vi "Save multiple images with metadata to new tiff stack.vi"(4 "ImageDescriptions":string[](array[string]), 5 "Add metadata? (T)":bool=TRUE, 6 "Show Progress? (T)":bool=TRUE, 7 "Compression Type (None)":i32(ring) items=["None", "JPEG", "Run Length Encoded", "Zip"], 8 "error in":errorcluster, 9 "Convert to U16?":bool, 10 "Array of Images (U8, U16, I16)":T1[](array[typedef]), 11 "Path":path) -> (0 "error out":errorcluster)   [LabVIEW 2013, in "Tiff reader.lvlib"]
doc: "This .vi saves an array of images into a new single .tiff stack file."
uses:
  Tiff reader.lvlib
  <vilib>/vision/Image Controls.llb/IMAQ Image.ctl
  <vilib>/vision/NI_Vision_Development_Module.lvlib
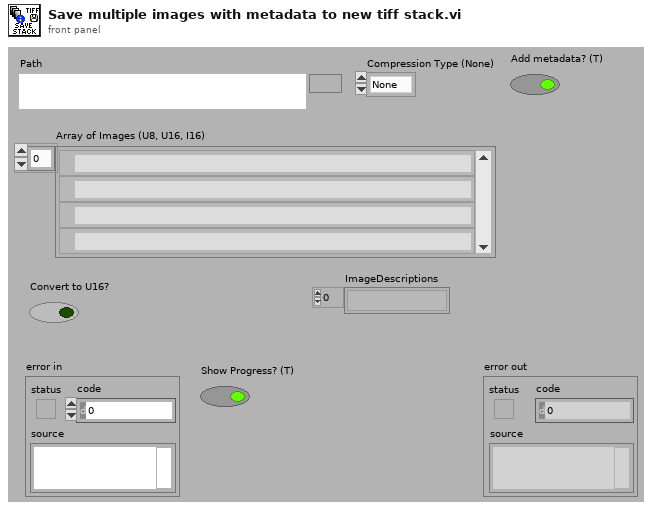
[diagram p1: front panel]
types:
  T1 = typedef "IMAQ Image.ctl" = refnum<image>
  T2 = cluster{"Rows Per Strip":i32, "Photometric":i32, "Compression Type":i32}
  T3 = typedef "Image Type" = u32
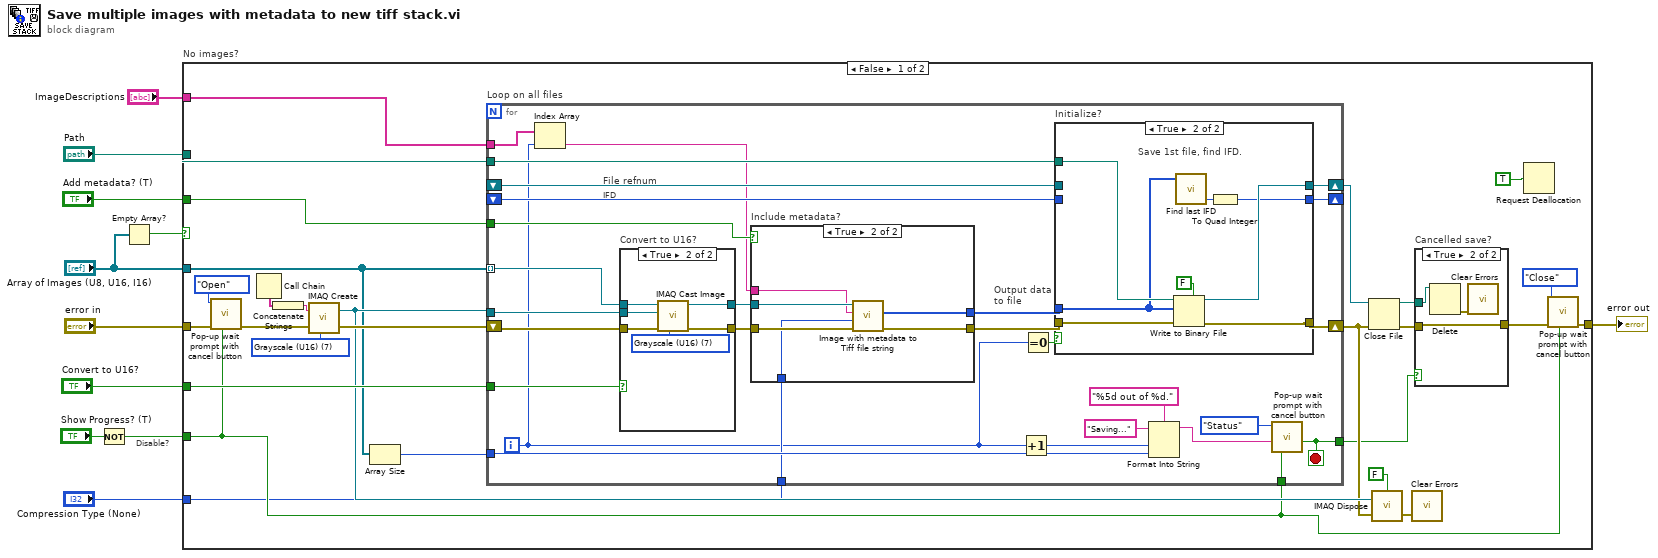
[diagram p0: block diagram]
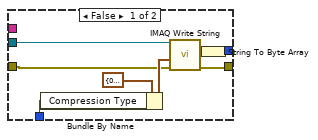
[diagram p3: hidden frame]
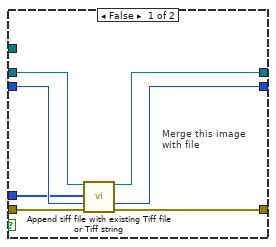
[diagram p5: hidden frame]
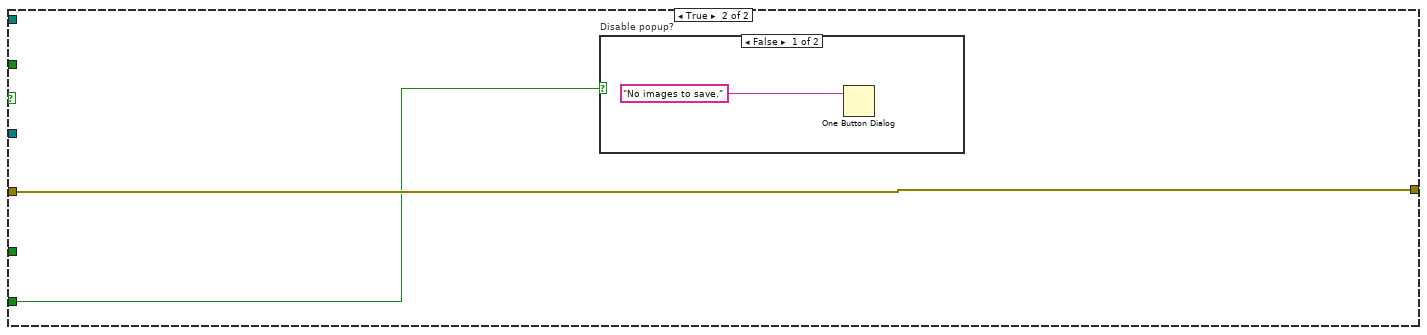
[diagram p6: hidden frame]
diagram:
  # "Disable?"
  n1 = Not(x="Show Progress? (T)") -> (.not. x?=w4:bool)
  n2 = Empty Array?(array="Array of Images (U8, U16, I16)") -> (empty?=w7:bool)
  n3 = case "No images?" shown="False" w7 {
    tunnel: "Array of Images (U8, U16, I16)" -> [w26 _]
    tunnel: [w38 w109] -> w10
    tunnel: "error in" -> [w35 w109]
    tunnel: "Path" -> [w31 _]
    tunnel: "Convert to U16?" -> [w28 _]
    tunnel: w4 -> [w17 w108]
    tunnel: "Compression Type (None)" -> [w16 _]
    tunnel: "Add metadata? (T)" -> [w14 _]
    tunnel: "ImageDescriptions" -> [w12 _]
    frame False {
      w30 = T3 7 items=["Grayscale (U8)", "Grayscale (I16)", "Grayscale (SGL)", "Complex (CSG)", "RGB (U32)", "HSL (U32)", "RGB (U64)", "Grayscale (U16)"] ("Image Type")
      n4 = call "Pop-up wait prompt with cancel button.vi"("Disable? (F)"=w17, "error in"=w35, "Control"=enum16{"Open", "Close", "Status", "No Change"}."Open") -> ("error out"=w20:errorcluster)  [unwired: 2 in, 6 out]
      n5 = Call Chain() -> (call chain=w19:string[])
      n6 = Concatenate Strings(w19) -> (w18:string)
      n7 = call "IMAQ Create"("Image Name"=w18, "Image Type"=w30, "error in (no error)"=w20) -> ("New Image"=w27:T1, "error out"=w29:errorcluster)  [unwired: 1 in, 1 out]
      n8 = Array Size(array=w26) -> (size(s)=w32:i32)
      n9 = for "Loop on all files" {
        tunnel: w26 -> [w57] mode=indexing
        tunnel: w31 -> [w69]
        shift-right: [w68] -> w23
        shift-left: w29 -> [w59]
        shift-right: [w67] -> w33
        shift-left: _ -> [w66]
        shift-right: [w64] -> _
        shift-left: _ -> [w65]
        tunnel: w32 -> [w61]
        tunnel: w27 -> [w58]
        tunnel: w28 -> [w56]
        tunnel: [w53] -> w22
        tunnel: w17 -> [w48]
        tunnel: w16 -> [w47]
        tunnel: w14 -> [w46]
        tunnel: w12 -> [w44]
        i -> [w45]
        stop <- w53 stop-if-true
        # "File refnum"
        # "IFD"
        # "Output data\nto file"
        n10 = Index Array(array=w44, index=w45) -> (element=w43:string)
        n11 = case "Convert to U16?" shown="True" w56 {
          tunnel: w59 -> [w85 w92]
          tunnel: [w85 w91] -> w51
          tunnel: w57 -> [w86 w90]
          tunnel: w58 -> [_ w89]
          tunnel: [w86 w87] -> w52
          frame False {
          }
          frame True {
            w88 = T3 7 items=["Grayscale (U8)", "Grayscale (I16)", "Grayscale (SGL)", "Complex (CSG)", "RGB (U32)", "HSL (U32)", "RGB (U64)", "Grayscale (U16)"] ("Image Type")
            n12 = call "IMAQ Cast Image"("Image Type"=w88, "error in (no error)"=w92, "Image Dst"=w89, "Image Src"=w90) -> ("error out"=w91:errorcluster, "Image Dst Out"=w87:T1)  [unwired: 2 in, 4 out]
          }
        }
        n13 = case "Include metadata?" shown="True" w46 {
          tunnel: w52 -> [w73 w84]
          tunnel: w51 -> [w74 w83]
          tunnel: [w75 w82] -> w50
          tunnel: [w71 w81] -> w49
          tunnel: w47 -> [w72 w80]
          tunnel: w43 -> [_ w79]
          frame False {
            n14 = Bundle By Name(cluster=T2 {"Rows Per Strip"=0, "Photometric"=1, "Compression Type"=0} ("TIFF Options"), "Compression Type"=w72) -> (w77:T2)
            n15 = call-poly "IMAQ Write String"("error in (no error)"=w74, "TIFF Options"=w77, "Image"=w73) -> ("error out"=w75:errorcluster, "FileString"=w76:string)  [unwired: 2 in, 5 out]
            n16 = String To Byte Array(string=w76) -> (unsigned byte array=w71:u8[])
          }
          frame True {
            n17 = call "Image with metadata to Tiff file string.vi"("error in"=w83, "Compression Type (None)"=w80, "ImageDescription string\n(must be at least 5 char long)"=w79, "img"=w84) -> ("error out"=w82:errorcluster, "Tiff file out (unsigned byte array)"=w81:u8[])  [unwired: 2 out]
          }
        }
        n18 = Increment(x=w45) -> (x+1=w60:i32)
        n19 = Equal To 0?(x=w45) -> (x = 0?=w70:bool)
        n20 = case "Initialize?" shown="True" w70 {
          tunnel: w50 -> [w98 w103]
          tunnel: w69 -> [_ w104]
          tunnel: [w99 w107] -> w68
          tunnel: [w96 w106] -> w67
          tunnel: w66 -> [w97 _]
          tunnel: w65 -> [w95 _]
          tunnel: [w94 w101] -> w64
          tunnel: w49 -> [w93 w100]
          frame False {
            # "Merge this image\nwith file"
            n21 = call "Append tiff file with existing Tiff file or Tiff string.vi"("Existing Tiff File (A) refnum"=w97, "Tiff file (B)\n (unsigned byte array)"=w93, "Location in existing file of\nit's last page's \n\"next IFD pointer\""=w95, "error in"=w98) -> ("File refnum out"=w96:refnum<file>, "Location in new file of\nit's last page's \n\"next IFD pointer\""=w94:i64, "error out"=w99:errorcluster)  [unwired: 3 in, 6 out]
          }
          frame True {
            # "Save 1st file, find IFD."
            n22 = Write to Binary File(file (use dialog)=w104, data=w100, error in=w103, 5:FALSE ("prepend array or string size? (T)")) -> (refnum out=w106:refnum<file>, error out=w107:errorcluster)  [unwired: 1 in, 2 out]
            n23 = call "Find last IFD.vi"("TIFF Data in"=w100) -> ("Location in byte stream of last IFD pointer.  This\nis the word to change if you are adding another page\nto the file."=w102:i32)  [unwired: 4 out]
            n24 = To Quad Integer(1:w102) -> (0:w101:i64)
          }
        }
        n25 = Format Into String(format string="%5d out of %d.", initial string="Saving..." ("Prompt Text"), w60, w61) -> (resulting string=w54:string)  [unwired: 1 in, 1 out]
        n26 = call "Pop-up wait prompt with cancel button.vi"("Disable? (F)"=w48, "Prompt Text"=w54, "Control"=enum16{"Open", "Close", "Status", "No Change"}."Status") -> ("Cancel"=w53:bool)  [unwired: 2 in, 6 out]
      }
      n27 = Close File(refnum=w33, error in=w23) -> (path=w24:path, error out=w25:errorcluster)
      n28 = call "IMAQ Dispose"("All Images? (No)"=FALSE, "Image"=w27, "error in (no error)"=w23) -> ("error out"=w34:errorcluster)  [unwired: 3 out]
      n29 = call <vilib>:"Clear Errors.vi"("error in (no error)"=w34) -> ()  [unwired: 7 out]
      n30 = case "Cancelled save?" shown="True" w22 {
        tunnel: w25 -> [w39 w40]
        tunnel: w24 -> [_ w42]
        tunnel: [w39 w40] -> w21
        frame False {
        }
        frame True {
          n31 = Delete(path (use dialog)=w42) -> (error out=w41:errorcluster)  [unwired: 1 in, 5 out]
          n32 = call <vilib>:"Clear Errors.vi"("error in (no error)"=w41) -> ()  [unwired: 7 out]
        }
      }
      n33 = Request Deallocation(TRUE ("flag")) -> ()
      n34 = call "Pop-up wait prompt with cancel button.vi"("Disable? (F)"=w17, "error in"=w21, "Control"=enum16{"Open", "Close", "Status", "No Change"}."Close") -> ("error out"=w38:errorcluster)  [unwired: 2 in, 6 out]
    }
    frame True {
      n35 = case "Disable popup?" shown="False" w108 {
        frame False {
          n36 = One Button Dialog(message="No images to save.") -> ()  [unwired: 2 out]
        }
        frame True {
        }
      }
    }
  }
  "error out" <- w10
